vi "Beat Blink.vi"() -> ()   [LabVIEW 2020]
uses:
  <vilib>/Platform/TimedLoop/XDataNode/timing_clust.ctl
  <vilib>/Platform/TimedLoop/XDataNode/nitl_modes.ctl
  <vilib>/Platform/TimedLoop/XDataNode/wakeup.ctl
  <vilib>/platform/TimedLoop/XDataNode/XDataNode.xnode
  <vilib>/Platform/TimedLoop/XDataNode/XDNodeRunTimeDep.lvlib
panel:
  in  "Phase [deg]":dbl=-90.0 min=-360.0 max=360.0 step=1.0
  out "Signal 2 [Hz]":dbl=0.5 step=0.01 format="%_3g"
  out "Signal 1 [Hz]":dbl=0.5 step=0.01 format="%_3g"
  out "Ratio":dbl=inf step=0.01
  out "Phasor diagram":cluster{dbl[], dbl[]}[](graph)=[{[0.0, 0.4086490747266945], [0.0, 0.9126915874078255]}, {[0.0, 0.9126915874078277], [0.0, -0.40864907472668954]}, {[0.0, 1.3213406621345223], [0.0, 0.504042512681136]}] caption="XY Graph"
  out "Sum of Signals":dbl(slide)=1.3213406621345223 scale=-2.0..2.0
  out "Individual Signals":waveform(dbl)(graph)={"t0"=timestamp(3695359275.707862 s since 1904-01-01), "dt"=0.002, "Y"=[1.3213406621345223]}
  out "Individual Signals":waveform(dbl)[](graph)=[{"t0"=timestamp(3695359275.707862 s since 1904-01-01), "dt"=0.002, "Y"=[0.4086490747266945]}, {"t0"=timestamp(3695359275.707862 s since 1904-01-01), "dt"=0.002, "Y"=[0.9126915874078277]}]
  in  "Difference [Hz]":dbl min=-1.0 max=1.0 step=0.01 format="%.2g"
  out "Individual Signals":cluster{dbl, dbl}(slide)={0.4086490747266945, 0.9126915874078277} scale=-2.0..2.0
  in  "Frequency [Hz]":dbl=0.5 min=0.0 max=10.0 step=0.05 format="%.2f"
  in  "Stop":bool
  # "Beat Signal Demo"
  # "McClellan et al., DSP First    \nCh. 3-2 Beat Notes"
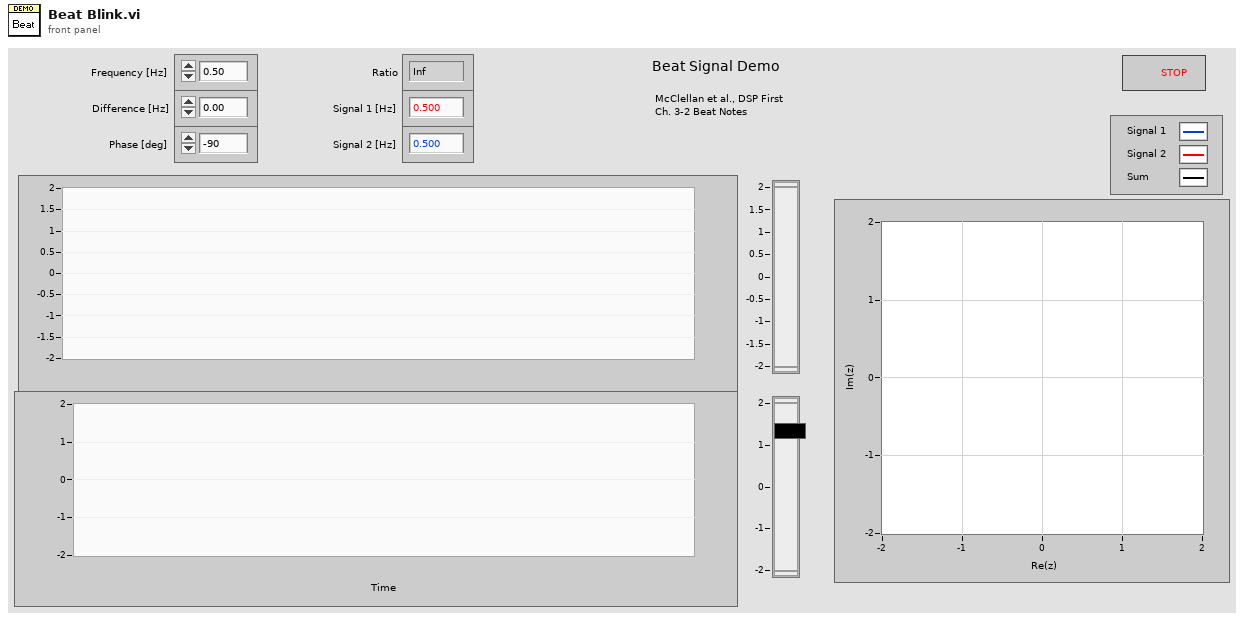
[diagram p1: front panel]
types:
  T1 = typedef "XDNodeRunTimeDep.lvlib/timing_clust.ctl" = cluster{"Expected End [f-1]":u64, "Actual End [f-1]":u64, "Finished Late? [f-1]":bool, "Expected End [i-1]":u64, "Actual End [i-1]":u64, "Finished Late? [i-1]":bool, "Expected Start [i]":u64, "Actual Start [i]":u64, "Expected Start [f]":u64, "Actual Start [f]":u64, "Source Name":string, "Structure Name":string, "Period":i64, "Deadline":i64, "Offset":i64, "Start":i64, "Priority":i32, "Timeout":i32, "Mode":T2, "Wakeup Reason":T3, "Error":errorcluster, "Source Type":string, "Secondary Source Type":string, "Global End Time":u64, "Global Start Time":u64, "Frame Duration":u64, "Iteration Duration":u64, "Assigned CPU":i32, "I/O Scan Engine Mode":u32}
  T2 = typedef "XDNodeRunTimeDep.lvlib/nitl_modes.ctl" = enum32{"No Change", "Process missed periods, maintain original phase", "Discard missed periods, maintain original phase", "Process missed periods, ignore original phase", "Discard missed periods, ignore original phase"}
  T3 = typedef "XDNodeRunTimeDep.lvlib/wakeup.ctl" = enum32{"Normal", "Aborted", "Asynchronous wakeup", "Timing source error", "Timed loop error", "Timeout"}
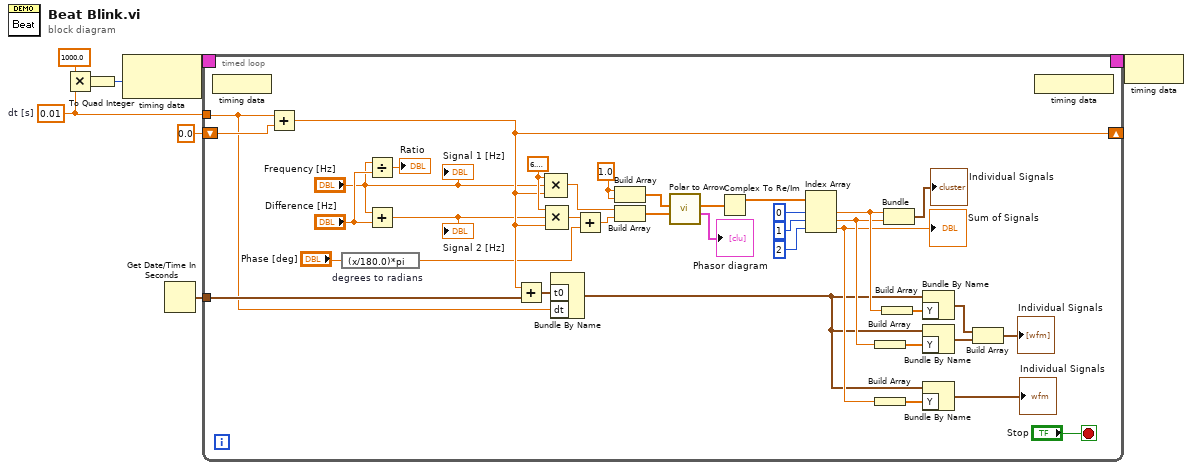
[diagram p0: block diagram]
diagram:
  w3 = 0.01  # dt [s]
  n1 = Multiply(x=1000.0 ("y"), y=w3) -> (x*y=w4:dbl)
  n2 = To Quad Integer(1:w4) -> (0:w2:i64)
  n3 = node-c288(w2) -> (w8:T1)
  n4 = Get Date/Time In Seconds() -> (seconds since 1Jan1904=w1:timestamp)
  n5 = timed-loop {
    timing: w8 -> [_]
    timing-out: [_] -> w7
    shift-right: [w39] -> _
    shift-left: 0.0 -> [w44]
    tunnel: w3 -> [w9]
    tunnel: w1 -> [w42]
    stop <- "Stop" stop-if-true
    w25 = 1.0 ("Magnitude")
    w43 = 6.283185307179586
    n6 = node-c288() -> ()  [unwired: 1 in]
    n7 = Add(x=w9, y=w44) -> (x+y=w39:dbl)
    n8 = expression code="(x/180.0)*pi" "degrees to radians"("Phase [deg]") -> (w16:dbl)
    n9 = Divide(x="Frequency [Hz]", y="Difference [Hz]") -> (x/y=→"Ratio":dbl)
    n10 = Add(x="Frequency [Hz]", y="Difference [Hz]") -> (x+y=w18:dbl)
    "Signal 2 [Hz]" <- w18
    n11 = Add(x=w39, y=w42) -> (x+y=w15:timestamp)
    n12 = Compound Arithmetic op=MULTIPLY(w43, "Frequency [Hz]", w39) -> (w38:dbl)
    n13 = Compound Arithmetic op=MULTIPLY(w43, w18, w39) -> (w21:dbl)
    n14 = Bundle By Name("t0"=w15, "dt"=w9) -> (w10:waveform(dbl))  [unwired: 1 in]
    n15 = Add(x=w21, y=w16) -> (x+y=w20:dbl)
    n16 = Build Array(w25, w25) -> (w26:dbl[])
    n17 = Build Array(w38, w20) -> (w37:dbl[])
    n18 = call "Polar to Arrow.vi"("Phases [rad]"=w37, "Magnitudes"=w26) -> ("Vector coordinates"=→"Phasor diagram":cluster{"Real":dbl[], "Imag":dbl[]}[], "z"=w35:cdb[])  [unwired: 7 in, 1 out]
    n19 = Complex To Re/Im(x + iy=w35) -> (x=w33:dbl[])  [unwired: 1 out]
    n20 = Index Array(array=w33, index #1=0 ("index"), index #2=1 ("index"), index #3=2 ("index")) -> (element #1=w30:dbl, element #2=w28:dbl, element #3=w24:dbl)
    "Sum of Signals" <- w24
    n21 = Build Array(w28) -> (w12:dbl[])
    n22 = Build Array(w24) -> (w27:dbl[])
    n23 = Build Array(w30) -> (w13:dbl[])
    n24 = Bundle("Numeric"=w30, "Numeric"=w28) -> (→"Individual Signals":cluster{"Numeric":dbl, "Numeric":dbl})  [unwired: 1 in]
    n25 = Bundle By Name(cluster=w10, "Y"=w13) -> (w14:waveform(dbl))
    n26 = Bundle By Name(cluster=w10, "Y"=w12) -> (w11:waveform(dbl))
    n27 = Bundle By Name(cluster=w10, "Y"=w27) -> (→"Individual Signals":waveform(dbl))
    n28 = Build Array(w14, w11) -> (→"Individual Signals":waveform(dbl)[])
    n29 = node-c288() -> ()  [unwired: 1 out]
    "Signal 1 [Hz]" <- "Frequency [Hz]"
  }
  n30 = node-c288(w7) -> ()
